vi "Example.vi"() -> ()   [LabVIEW 2019, in "Modbus DataType Conversation.lvlib"]
uses:
  Modbus DataType Conversation.lvlib
  SGL to U16.vi
panel:
  out "REGs U16":u16[](array[numeric])
  out "SGL out":sgl[](array[numeric])
  in  "SGL in":sgl[](array[numeric])=[1.1, 2.2, 3.3]
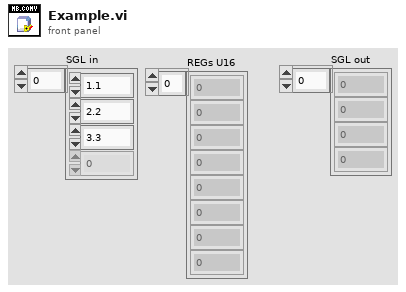
[diagram p1: front panel]
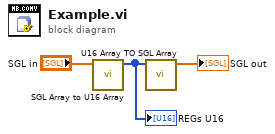
[diagram p0: block diagram]
diagram:
  n1 = call "SGL Array to U16 Array.vi"("SGL"="SGL in") -> ("REG U16"=w3:u16[])  [unwired: 10 in]
  "REGs U16" <- w3
  n2 = call "U16 Array TO SGL Array.vi"("REG U16"=w3) -> ("SGL"=→"SGL out":sgl[])  [unwired: 10 in]
